vi "To String.vi"(8 "error in":errorcluster, 11 "CAN Message in":refnum<class "CAN Message.lvclass">) -> (0 "error out":errorcluster, 2 "Stringified":string, 3 "CAN Message out":refnum<class "CAN Message.lvclass">)   [LabVIEW 2024, in "CAN Message.lvclass"]
uses:
  CAN Message.lvclass
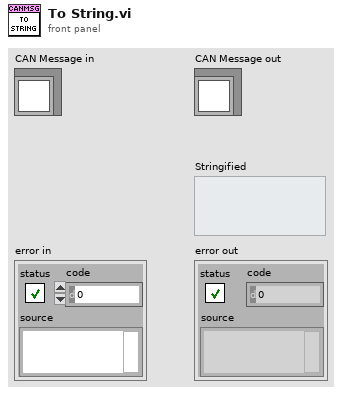
[diagram p1: front panel]
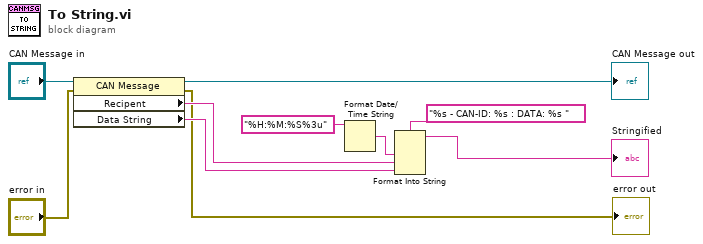
[diagram p0: block diagram]
diagram:
  n1 = property class="CAN Message"(reference="CAN Message in", error in="error in") -> (reference out=→"CAN Message out":refnum<class "CAN Message.lvclass">, error out=→"error out":errorcluster, "Recipent"=w5:string, "Data String"=w4:string)
  n2 = Format Date/Time String(time format string (%c)="%H:%M:%S%3u") -> (date/time string=w2:string)  [unwired: 2 in]
  n3 = Format Into String(format string="%s - CAN-ID: %s : DATA: %s ", w2, w5, w4) -> (resulting string=→"Stringified":string)  [unwired: 2 in, 1 out]
